vi "Table Stage GUI.vi"() -> ()   [LabVIEW 2014]
uses:
  Hardware/Table Stage/Controls/Translation Stage Cluster.ctl
  Controls/Translation Stage Types.ctl
  Controls/Queue Manager Actions.ctl
  Controls/QueueNames.ctl
  Controls/MessagePacket.ctl
  Controls/Table Stage GUI Front Panel Configurator AFGV Actions.ctl
  Hardware/Table Stage/Controls/Motion Translation Module Control.ctl
  Controls/FGV Actions.ctl
panel:
  in  "Save and Connect":bool
  in  "Close":bool
  in  "Tab Control":enum32{"Page 1"}(tab)
  out "Z":bool
  in  "X Position 4":dbl caption="Z"
  out "Y":bool
  in  "X Position 3":dbl caption="Y"
  out "X":bool
  in  "X Position":dbl caption="X"
  in  "dX 4":dbl caption="Increment"
  in  "-X":bool
  in  "+X":bool
  in  "dX 3":dbl caption="Increment"
  in  "Previous Button":bool
  in  "Next Button":bool
  in  "Down Button":bool
  in  "Up Button":bool
  in  "Stop":bool
  in  "Reconnect":bool
  in  "Home Stages":bool
  in  "Identify":bool
  in  "Axis":enum16{"X Axis", "Y Axis", "Z Axis"}(ring)
  in  "Show Advanced":bool
  in  "Cluster In 3":T1={"Position"=0.0, "Is.Enabled?"=TRUE, "Is.Connected?"=FALSE, "Device SN"="45876539", "AccelerationMaximum"=0.0, "VelocityMaximum"=0.0, "Acceleration"=0.0, "Velocity"=0.0, "waitTimeout (ms)"=10000, "Model"=enum."None", "Is.Homed?"=FALSE}
  in  "Controller Information":T1={"Position"=0.0, "Is.Enabled?"=TRUE, "Is.Connected?"=FALSE, "Device SN"="45876539", "AccelerationMaximum"=0.0, "VelocityMaximum"=0.0, "Acceleration"=0.0, "Velocity"=0.0, "waitTimeout (ms)"=10000, "Model"=enum."None", "Is.Homed?"=FALSE}
  out "Error Out":errorcluster
  in  "Error In":errorcluster
  # "XYZ TABLE STAGE CONTROLS"
  # "Position"
  # "Enable"
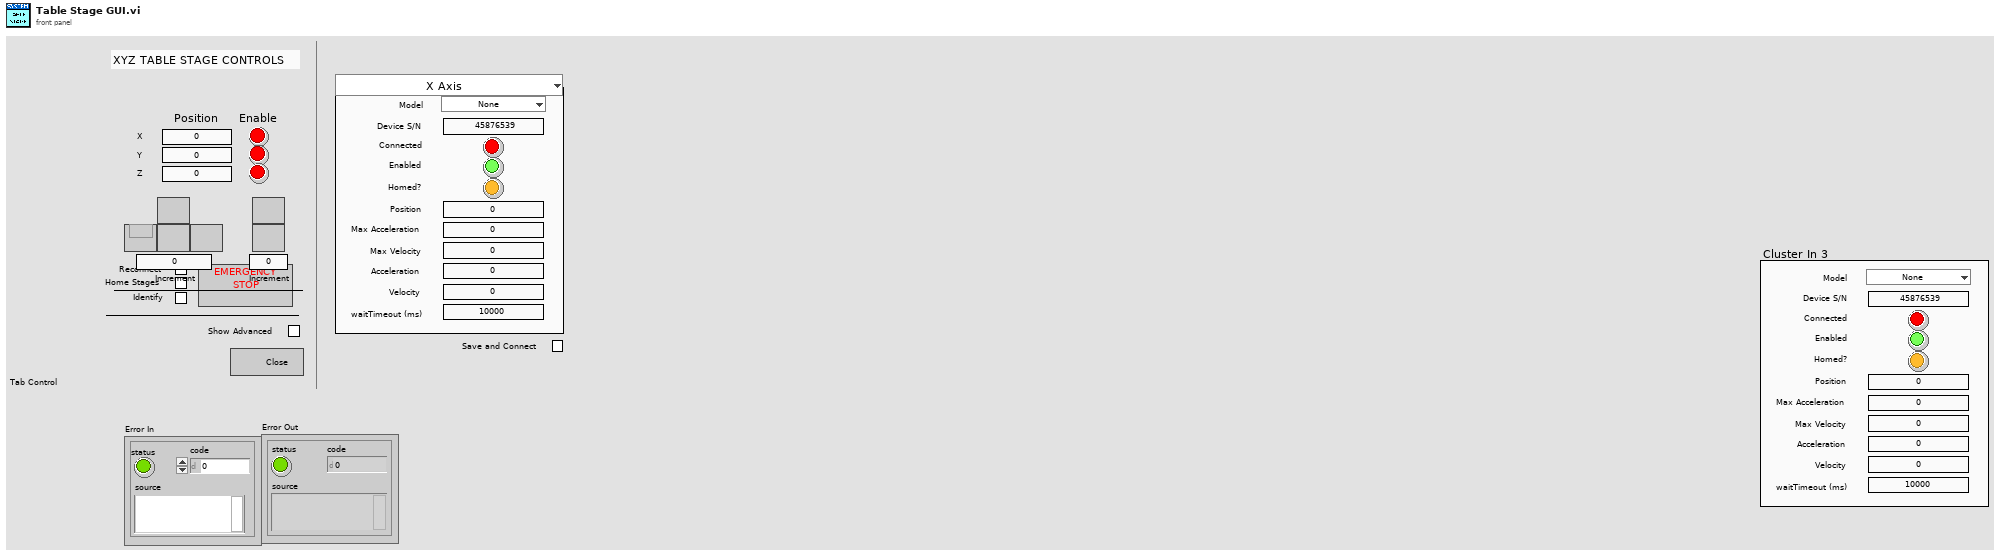
[diagram p1: front panel]
types:
  T1 = typedef "Translation Stage Cluster.ctl" = cluster{"Position":dbl, "Is.Enabled?":bool, "Is.Connected?":bool, "Device SN":string, "AccelerationMaximum":dbl, "VelocityMaximum":dbl, "Acceleration":dbl, "Velocity":dbl, "waitTimeout (ms)":i32, "Model":T2, "Is.Homed?":bool}
  T2 = typedef "Translation Stage Types.ctl" = enum16{"None", "Thorlabs LTS", "Thorlabs MLJ"}
  T3 = typedef "MessagePacket.ctl" = cluster{"Message":string, "Parameter":variant}
  T4 = typedef "QueueNames.ctl" = enum16{"Main GUI", "Main Scan Processor", "Main Display", "Main Table Stage GUI", "Main Table Stage Proc.", "Scan Engine"}
  T5 = typedef "Queue Manager Actions.ctl" = enum16{"Init", "Enqueue", "Enqueue All", "Preview Queue", "Dequeue", "Get Status", "Flush Queue", "Flush All Queues", "Release All Queues", "Release Queue", "Enqueue at Opposite End"}
  T6 = typedef "FGV Actions.ctl" = enum16{"Init", "Set", "Get", "Clear"}
  T7 = typedef "Motion Translation Module Control.ctl" = enum16{"Init", "Home", "Configure", "Velocity/Accel", "Position", "Jog", "Stop", "Uninit"}
  T8 = typedef "Table Stage GUI Front Panel Configurator AFGV Actions.ctl" = enum16{"Init", "Defer FP Update", "Enable FP Update", "Disable Ctrls", "Enable Ctrls", "Basic", "Advanced"}
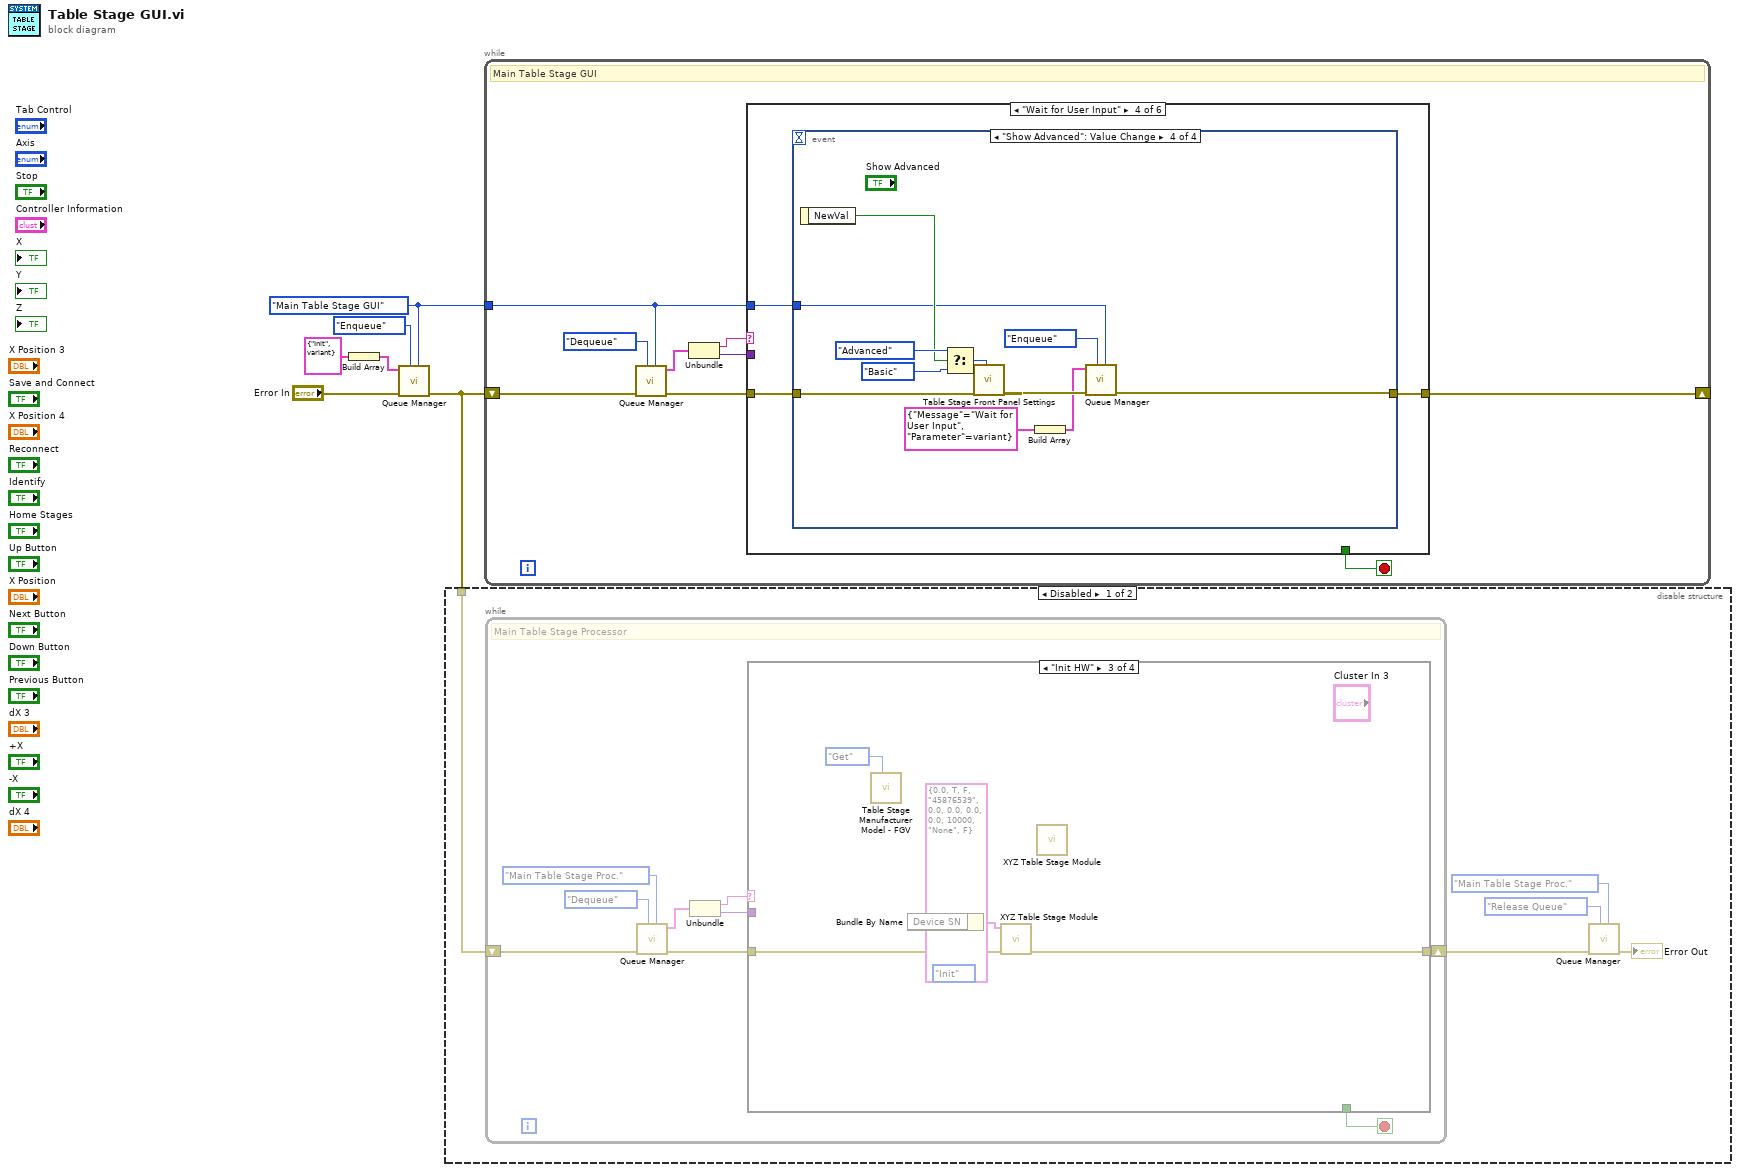
[diagram p0: block diagram]
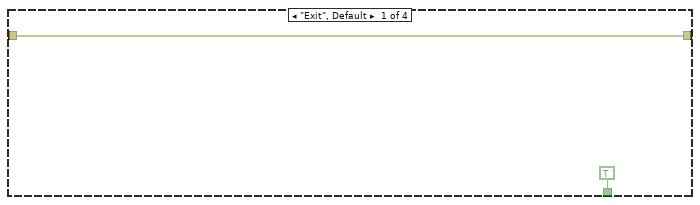
[diagram p2: hidden frame]
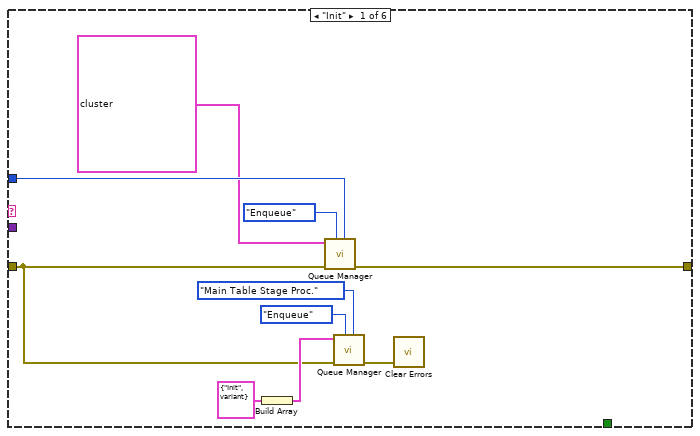
[diagram p6: hidden frame]
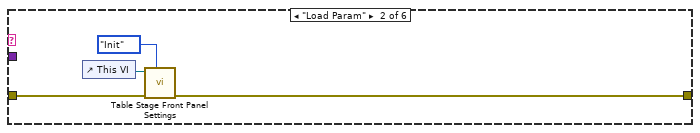
[diagram p7: hidden frame]
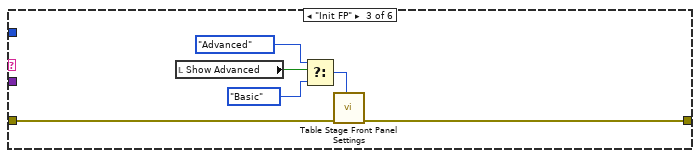
[diagram p8: hidden frame]
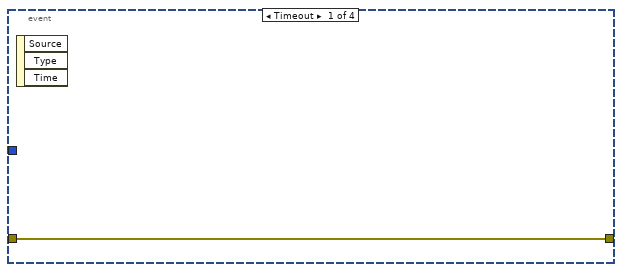
[diagram p9: hidden frame]
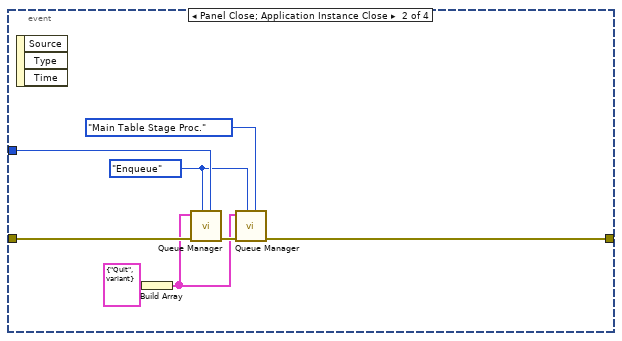
[diagram p10: hidden frame]
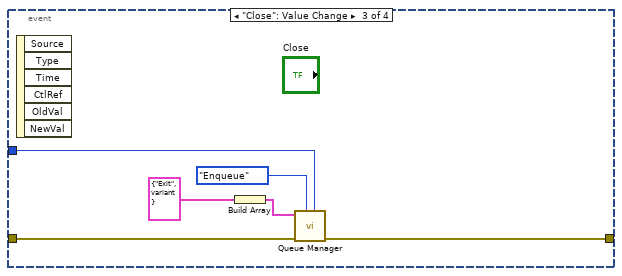
[diagram p11: hidden frame]
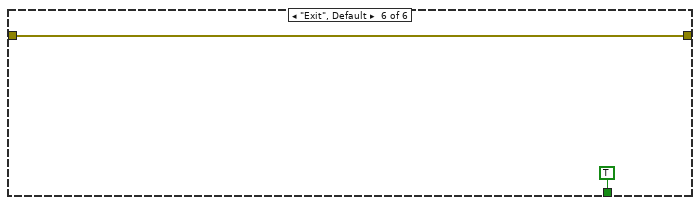
[diagram p13: hidden frame]
diagram:
  w1 = QueueNames."Main Table Stage GUI" ("Queue Name")
  n1 = Build Array(T3 {"Message"="Init", "Parameter"=variant} ("Message Packet [In]")) -> (w2:T3[])
  n2 = call "Queue Manager.vi"("Queue Name"=w1, "Action"=Queue_Manager_Actions."Enqueue", "Error In"="Error In", "Message Packet Array"=w2) -> ("Error Out"=w4:errorcluster)  [unwired: 5 in, 2 out]
  n3 = disable-structure shown="Disabled" {
    disable-tunnel: w4 -> [w7 _]
    frame Disabled {
      n4 = while {
        shift-right: [w13] -> w11
        shift-left: w7 -> [w18]
        stop <- w12 stop-if-true
        # "Main Table Stage Processor"
        n5 = call "Queue Manager.vi"("Queue Name"=QueueNames."Main Table Stage Proc.", "Action"=Queue_Manager_Actions."Dequeue", "Error In"=w18) -> ("Error Out"=w17:errorcluster, "Message Packet [Out]"=w16:T3)  [unwired: 6 in, 1 out]
        n6 = Unbundle(w16) -> ("Message"=w15:string, "Parameter"=w14:variant)
        n7 = case shown="\"Init HW\"" w15 {
          tunnel: w17 -> [w21 w23 w27 w30]
          tunnel: w14 -> [_ _ _ _]
          tunnel: [w21 w23 w26 w30] -> w13
          tunnel: [TRUE _ _ _] -> w12
          frame "Exit", Default {
          }
          frame "Init" {
          }
          frame "Init HW" {
            (unwired) Motion_Translation_Module_Control."Init" ("Action")
            n8 = call "Table Stage Manufacturer Model - FGV.vi"("Actions"=FGV_Actions."Get") -> ()  [unwired: 9 in, 2 out]
            n9 = Bundle By Name(cluster=T1 {"Position"=0.0, "Is.Enabled?"=TRUE, "Is.Connected?"=FALSE, "Device SN"="45876539", "AccelerationMaximum"=0.0, "VelocityMaximum"=0.0, "Acceleration"=0.0, "Velocity"=0.0, "waitTimeout (ms)"=10000, "Model"=enum."None", "Is.Homed?"=FALSE} ("Cluster In")) -> (w25:T1, "Device SN"=w28:string)
            n10 = call "XYZ Table Stage Module.vi"("Error In"=w27, "Control Param In"=w25) -> ("Error Out"=w26:errorcluster)  [unwired: 9 in]
            n11 = call "XYZ Table Stage Module.vi"() -> ()  [unwired: 11 in, 1 out]
          }
          frame "Idle" {
          }
        }
      }
      n12 = call "Queue Manager.vi"("Queue Name"=QueueNames."Main Table Stage Proc.", "Action"=Queue_Manager_Actions."Release Queue", "Error In"=w11) -> ("Error Out"=→"Error Out":errorcluster)  [unwired: 6 in, 2 out]
    }
    frame Enabled {
    }
  }
  n13 = while {
    shift-right: [w32] -> _
    shift-left: w4 -> [w38]
    tunnel: w1 -> [w31]
    stop <- w33 stop-if-true
    # "Main Table Stage GUI"
    n14 = call "Queue Manager.vi"("Queue Name"=w31, "Action"=Queue_Manager_Actions."Dequeue", "Error In"=w38) -> ("Error Out"=w37:errorcluster, "Message Packet [Out]"=w36:T3)  [unwired: 6 in, 1 out]
    n15 = Unbundle(w36) -> ("Message"=w35:string, "Parameter"=w34:variant)
    n16 = case shown="\"Wait for User Input\"" w35 {
      tunnel: w37 -> [w43 w51 w59 w62 w89 w90]
      tunnel: w34 -> [_ _ _ _ _ _]
      tunnel: [w45 w50 w58 w61 w89 w90] -> w32
      tunnel: [_ _ _ _ _ TRUE] -> w33
      tunnel: w31 -> [w42 _ _ w60 _ _]
      frame "Init" {
        n17 = Build Array(T3 {"Message"="Init", "Parameter"=variant} ("Message Packet [In]")) -> (w46:T3[])
        n18 = call "Queue Manager.vi"("Queue Name"=w42, "Action"=Queue_Manager_Actions."Enqueue", "Error In"=w43, "Message Packet Array"=T3[] [{"Message"="Load Param", "Parameter"=variant}, {"Message"="Init FP", "Parameter"=variant}, {"Message"="Wait for User Input", "Parameter"=variant}]) -> ("Error Out"=w45:errorcluster)  [unwired: 5 in, 2 out]
        n19 = call "Queue Manager.vi"("Queue Name"=QueueNames."Main Table Stage Proc.", "Action"=Queue_Manager_Actions."Enqueue", "Error In"=w43, "Message Packet Array"=w46) -> ("Error Out"=w44:errorcluster)  [unwired: 5 in, 2 out]
        n20 = call <vilib>:"Clear Errors.vi"("error in (no error)"=w44) -> ()  [unwired: 5 in, 2 out]
      }
      frame "Load Param" {
        n21 = control-ref of="This VI"() -> (w53:refnum<vi>)
        n22 = call "Table Stage Front Panel Settings.vi"("Actions"=Table_Stage_GUI_Front_Panel_Configurator_AFGV_Actions."Init", "Error In"=w51, "This VI"=w53) -> ("Error Out"=w50:errorcluster)  [unwired: 8 in]
      }
      frame "Init FP" {
        n23 = local read "Show Advanced"() -> (w57:bool)
        n24 = Select(t=Table_Stage_GUI_Front_Panel_Configurator_AFGV_Actions."Advanced" ("Actions"), s=w57, f=Table_Stage_GUI_Front_Panel_Configurator_AFGV_Actions."Basic" ("Actions")) -> (s? t:f=w54:T8)
        n25 = call "Table Stage Front Panel Settings.vi"("Actions"=w54, "Error In"=w59) -> ("Error Out"=w58:errorcluster)  [unwired: 9 in]
      }
      frame "Wait for User Input" {
        n26 = event shown="[3] \"Show Advanced\": Value Change" {
          selector: _ -> [_ _ _ _]
          dyn-events: _ -> [_ _ _ _]
          timeout: _ -> [_ _ _ _]
          tunnel: w62 -> [w63 w71 w77 w85]
          tunnel: [w63 w67 w76 w82] -> w61
          tunnel: w60 -> [_ w70 w75 w81]
          event Timeout {
            n27 = event-data() -> ()  [unwired: 1 in, 3 out]
          }
          event Panel Close; Application Instance Close {
            w65 = Queue_Manager_Actions."Enqueue" ("Action")
            n28 = event-data() -> ()  [unwired: 1 in, 3 out]
            n29 = Build Array(T3 {"Message"="Quit", "Parameter"=variant} ("Message Packet [In]")) -> (w66:T3[])
            n30 = call "Queue Manager.vi"("Queue Name"=w70, "Action"=w65, "Error In"=w71, "Message Packet Array"=w66) -> ("Error Out"=w68:errorcluster)  [unwired: 5 in, 2 out]
            n31 = call "Queue Manager.vi"("Queue Name"=QueueNames."Main Table Stage Proc.", "Action"=w65, "Error In"=w68, "Message Packet Array"=w66) -> ("Error Out"=w67:errorcluster)  [unwired: 5 in, 2 out]
          }
          event "Close": Value Change {
            n32 = event-data() -> ()  [unwired: 1 in, 6 out]
            n33 = Build Array(T3 {"Message"="Exit", "Parameter"=variant} ("Message Packet [In]")) -> (w72:T3[])
            n34 = call "Queue Manager.vi"("Queue Name"=w75, "Action"=Queue_Manager_Actions."Enqueue", "Error In"=w77, "Message Packet Array"=w72) -> ("Error Out"=w76:errorcluster)  [unwired: 5 in, 2 out]
          }
          event "Show Advanced": Value Change {
            n35 = event-data() -> ("NewVal"=w83:bool)  [unwired: 1 in]
            n36 = Select(t=Table_Stage_GUI_Front_Panel_Configurator_AFGV_Actions."Advanced" ("Actions"), s=w83, f=Table_Stage_GUI_Front_Panel_Configurator_AFGV_Actions."Basic" ("Actions")) -> (s? t:f=w86:T8)
            n37 = call "Table Stage Front Panel Settings.vi"("Actions"=w86, "Error In"=w85) -> ("Error Out"=w84:errorcluster)  [unwired: 9 in]
            n38 = Build Array(T3 {"Message"="Wait for User Input", "Parameter"=variant} ("Message Packet [In]")) -> (w78:T3[])
            n39 = call "Queue Manager.vi"("Queue Name"=w81, "Action"=Queue_Manager_Actions."Enqueue", "Error In"=w84, "Message Packet Array"=w78) -> ("Error Out"=w82:errorcluster)  [unwired: 5 in, 2 out]
          }
        }
      }
      frame "Idle" {
      }
      frame "Exit", Default {
      }
    }
  }
